vi "EventLog.Gui.vi"() -> ()   [LabVIEW 2016]
uses:
  <vilib>/Utility/miscctls.llb/LVRowAndColumnUnsignedTypeDef.ctl
  Global/ApplicationGlobal.vi
  Config/Config.Global.vi
  Translator/Translator.Global.vi
panel:
  out "Panel":refnum<vi>
  out "_loop":i32(ring)=4
  out "Events":i32(listbox)
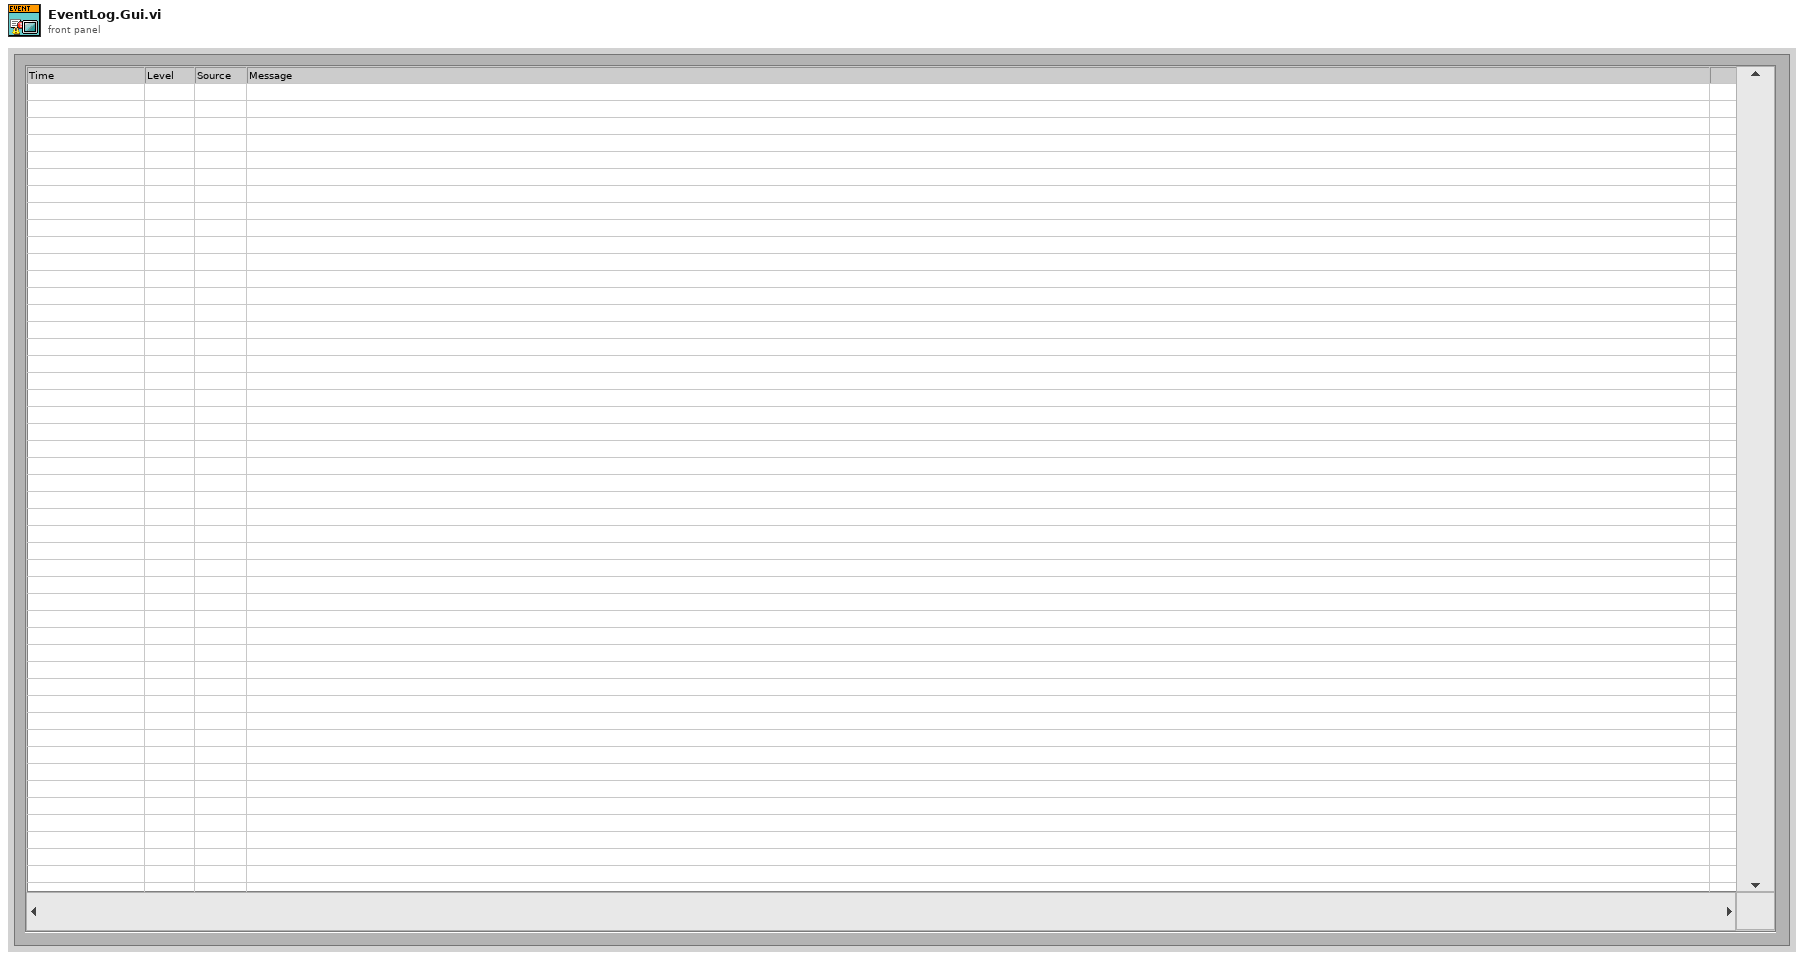
[diagram p1: front panel]
types:
  T1 = typedef "LVRowAndColumnUnsignedTypeDef.ctl" = cluster{"Row":u32, "Column":u32}
  T2 = typedef "LVPositionTypeDef.ctl" = cluster{"Left":i32, "Top":i32}
  T3 = typedef "EventLog.Gui.Sets.ctl" = cluster{"IncludeBegin":bool, "dtm_Begin":timestamp, "IncludeEnd":bool, "dtm_End":timestamp, "Events Level Operator":T4, "Level":u16, "Source":u16, "SearchText":string, "Freeze":bool}
  T4 = typedef "EventLog.EventLevelOperatorGui.ctl" = enum16{">=", "=", "<="}
  T5 = enum32{"Invalid", "Standard", "Closed", "Hidden", "Minimized", "Maximized"}
  T6 = typedef "EventLog.EventGui.ctl" = cluster{"ts":dbl, "lev":T7, "src":T8, "msg":T9, "arg":variant[], "msg_str":string}
  T7 = typedef "EventLog.EventLevel.ctl" = enum8{"Debug", "Info", "Warning", "Error"}
  T8 = typedef "EventLog.EventSource.ctl" = enum16{"All", "Gui", "PLC1", "PLC2", "PLC3", "DB", "DB01", "DB02", "DB03", "DB04", "DB05", "DB06", "DB07", "DB08", "DB09", "DB10", "DB11", "DB12", "DB13", "DB14", "DB15", "DB16"}
  T9 = typedef "Translator.Message.ctl" = enum16{"-", "Event confirmed", "Log out", "Log in", "Shutdown", "Cancel", "Start", "Continue", "Stop", "On", "Off", "OK", "NOK", "NOK %s", "This", "Prev", "Home", "Work", "In progress...", "Missing", "Empty", "Hardware failure", "Initial", "Error %d >> %s", "Error %d >> %s >> %s", "Starting %s", "Quitting %s", "Configured", "Initializing", "Quitting", "Loading", "Running %s", "Stopped", "Summary", "Do you want to continue?", "Do you want to exit?", "Log out?", "System", "All", "IDLE", "Translating...%s", "Not found", "Alarm %s", "Run", "Skip", "Abort", "Repeat", "Please wait...", "Database disconnected", "Login to database successful", "Login to database failed: %d; %s", "Get process step data for %s", "Changeover off", "Changeover into %s", "Product %s | %s found in cache with status %d at previous station", "Product %s | %s found in database with status %d at previous station", "Product %s | %s not found in cache at previous station", "Product %s | %s not found in database at previous station", "Product %s | %s found in cache with status %d at this station (%d repetion)", "Product %s | %s found in database with status %d at this station (%d repetition)", "Product %s | %s not found in cache at this station", "Product %s | %s not found in database at this station", "Product %s | %s found in cache for component %s | %s", "Product %s | %s found in database for component %s | %s", "Product not found in cache for component %s | %s", "Product not found in database for component %s | %s", "Product %s | %s connected with component %s | %s (cache)", "Product %s | %s connected with component %s | %s (database)", "New data for %s | %s (cache)", "New data for %s | %s (database)", "Msg %d >> %s", "PLC LifeBit Failure", "Reconnecting DB", "Reconnecting PLC"}
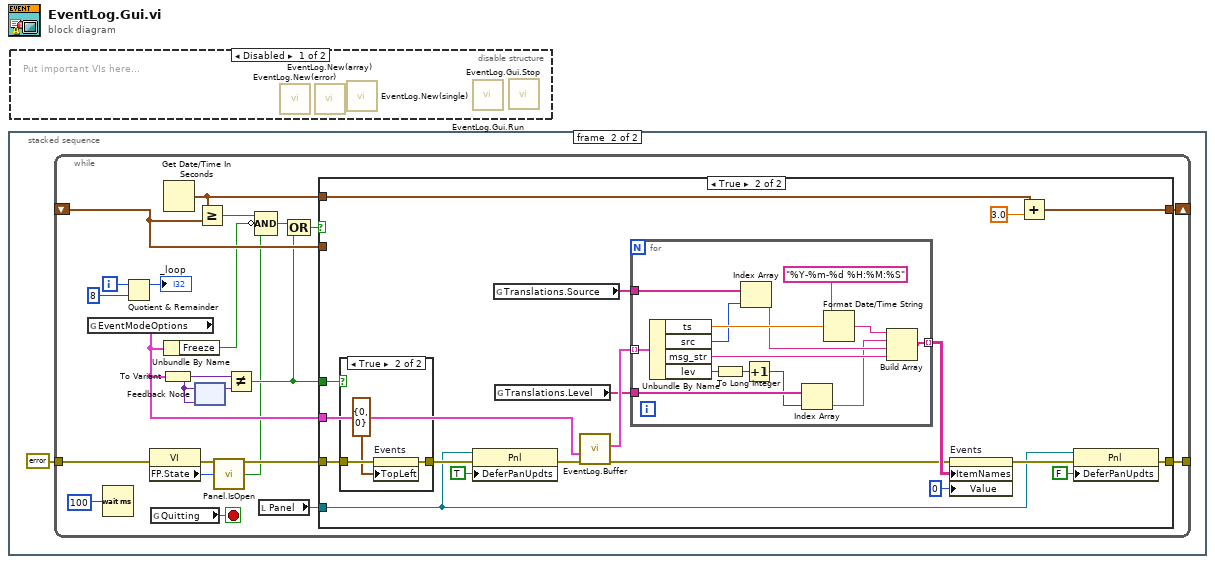
[diagram p0: block diagram]
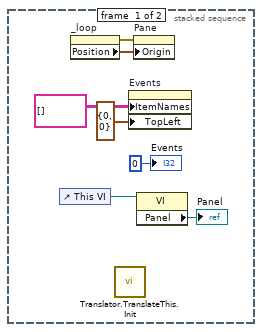
[diagram p2: hidden frame]
diagram:
  n1 = stacked-sequence {
    frame #0 {
      n2 = control-ref of="This VI"() -> (w2:refnum<vi>)
      n3 = property on="_loop" class="Ring (strict)"() -> (error out=w7:errorcluster, "Position"=w6:T2)  [unwired: 2 in, 1 out]
      n4 = call "Translator.TranslateThis.Init.vi"() -> ()  [unwired: 11 in, 1 out]
      n5 = property on="Events" class="MCListbox (strict)"("ItemNames"=string[][] [] ("Item Names"), "TopLeft"=T1 {"Row"=0, "Column"=0} ("Top Left Visible Cell")) -> ()  [unwired: 2 in, 2 out]
      n6 = property on="Pane" class="Pane"(error in=w7, "Origin"=w6) -> ()  [unwired: 1 in, 2 out]
      n7 = property class="VI"(reference=w2) -> ("Panel"=→"Panel":refnum<vi>)  [unwired: 1 in, 2 out]
      "Events" <- 0 ("Events")
    }
    frame #1 {
      n8 = while {
        shift-right: [w30] -> _
        shift-left: _ -> [w29]
        tunnel: errorcluster {"status"=FALSE, "code"=0, "source"=""} ("error out") -> [w27]
        tunnel: [w28] -> _
        i -> [w13]
        stop <- w25 stop-if-true
        n9 = global read "Config.Global.vi" "EventModeOptions"() -> (w24:T3)
        n10 = Wait (ms)(milliseconds to wait=u32 100) -> ()  [unwired: 1 out]
        n11 = Quotient & Remainder(x=w13, y=8) -> (x-y*floor(x/y)=→"_loop":i32)  [unwired: 1 out]
        n12 = property class="VI"(error in=w27) -> (error out=w26:errorcluster, "FP.State"=w10:T5)  [unwired: 1 in, 1 out]
        n13 = global read "ApplicationGlobal.vi" "Quitting"() -> (w25:bool)
        n14 = To Variant(anything=w24) -> (Variant=w19:variant)
        n15 = Get Date/Time In Seconds() -> (seconds since 1Jan1904=w21:timestamp)
        n16 = Unbundle By Name(w24) -> ("Freeze"=w20:bool)
        n17 = feedback #1(w19) -> (w18:variant)
        n18 = feedback-in #1(w19) -> ()
        n19 = Greater Or Equal?(x=w21, y=w29) -> (x >= y?=w23:bool)
        n20 = call "Panel.IsOpen.vi"("FP State"=w10) -> ("Open?"=w9:bool)
        n21 = Not Equal?(x=w19, y=w18) -> (x != y?=w16:bool)
        n22 = Compound Arithmetic op=AND(w23, invert w20, w9) -> (w22:bool)
        n23 = local read "Panel"() -> (w11:refnum<vi>)
        n24 = Compound Arithmetic op=OR(w22, w16) -> (w15:bool)
        n25 = case shown="True" w15 {
          tunnel: w26 -> [w32 w42]
          tunnel: [w32 w33] -> w28
          tunnel: [w31 w47] -> w30
          tunnel: w21 -> [_ w46]
          tunnel: w29 -> [w31 _]
          tunnel: w24 -> [_ w40]
          tunnel: w16 -> [_ w41]
          tunnel: w11 -> [_ w35]
          frame False {
          }
          frame True {
            n26 = case shown="True" w41 {
              tunnel: w42 -> [w52 w55]
              tunnel: [w52 w54] -> w38
              frame False {
              }
              frame True {
                n27 = property on="Events" class="MCListbox (strict)"(error in=w55, "TopLeft"=T1 {"Row"=0, "Column"=0} ("Top Left Visible Cell")) -> (error out=w54:errorcluster)  [unwired: 1 in, 1 out]
              }
            }
            n28 = property class="Pnl"(reference=w35, error in=w38, "DeferPanUpdts"=TRUE ("Defer Panel Updates")) -> (error out=w37:errorcluster)  [unwired: 1 out]
            n29 = global read "Translator.Global.vi" "Translations.Source"() -> (w43:string[])
            n30 = global read "Translator.Global.vi" "Translations.Level"() -> (w50:string[])
            n31 = call "EventLog.Buffer.vi"("error in"=w37, "Event.Sets"=w40) -> ("error out"=w48:errorcluster, "data out"=w51:T6[])  [unwired: 6 in, 2 out]
            n32 = for {
              tunnel: [w67] -> w49 mode=indexing
              tunnel: w51 -> [w66] mode=indexing
              tunnel: w50 -> [w64]
              tunnel: w43 -> [w60]
              n33 = Unbundle By Name(w66) -> ("ts"=w68:dbl, "src"=w58:T8, "msg_str"=w63:string, "lev"=w62:T7)
              n34 = To Long Integer(number=w62) -> (32bit integer=w57:i32)
              n35 = Index Array(array=w60, index=w58) -> (element=w59:string)
              n36 = Increment(x=w57) -> (x+1=w61:i32)
              n37 = Index Array(array=w64, index=w61) -> (element=w56:string)
              n38 = Format Date/Time String(time format string (%c)="%Y-%m-%d %H:%M:%S", seconds (now)=w68) -> (date/time string=w65:string)  [unwired: 1 in]
              n39 = Build Array(w65, w56, w59, w63) -> (w67:string[])
            }
            n40 = property on="Events" class="MCListbox (strict)"(error in=w48, "ItemNames"=w49, "Value"=0 ("Events")) -> (error out=w36:errorcluster)  [unwired: 1 in, 1 out]
            n41 = Add(x=w46, y=3.0) -> (x+y=w47:timestamp)
            n42 = property class="Pnl"(reference=w35, error in=w36, "DeferPanUpdts"=FALSE ("Defer Panel Updates")) -> (error out=w33:errorcluster)  [unwired: 1 out]
          }
        }
      }
    }
  }
  n43 = disable-structure shown="Disabled" {
    frame Disabled {
      # "Put important VIs here..."
      n44 = call "EventLog.New(error).vi"() -> ()  [unwired: 11 in, 1 out]
      n45 = call "EventLog.New(array).vi"() -> ()  [unwired: 10 in, 2 out]
      n46 = call "EventLog.New(single).vi"() -> ()  [unwired: 10 in, 2 out]
      n47 = call "EventLog.Gui.Run.vi"() -> ()  [unwired: 10 in, 2 out]
      n48 = call "EventLog.Gui.Stop.vi"() -> ()  [unwired: 11 in, 1 out]
    }
    frame Enabled {
    }
  }
